vi "ProceduralControlSystem.vi"() -> ()   [LabVIEW 2021]
panel:
  out "Solenoid Outputs":bool[](array[boolean])
  in  "Sensor Values":dbl[](array[numeric])
  in  "File Path":path[](array[path])
  in  "Dry Test Run":bool
  in  "Ignition":bool
  in  "Mainain Pressure":bool
  in  "Device & Valve Diagnostics":bool[](array[boolean])
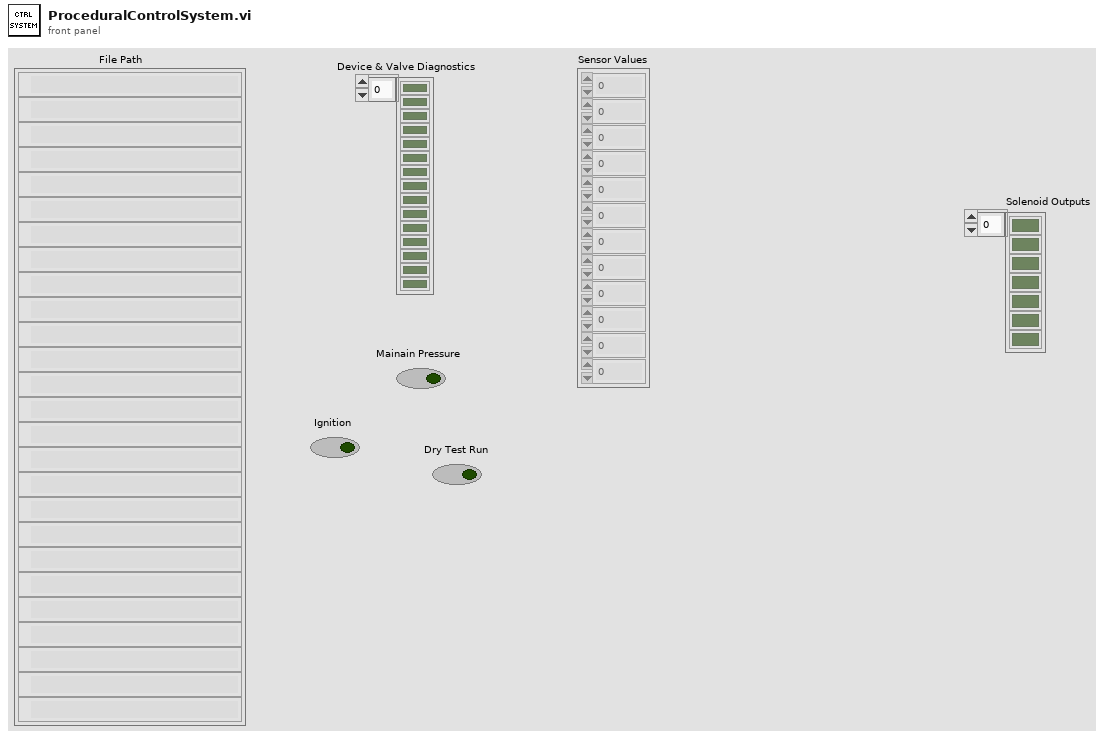
[diagram p1: front panel]
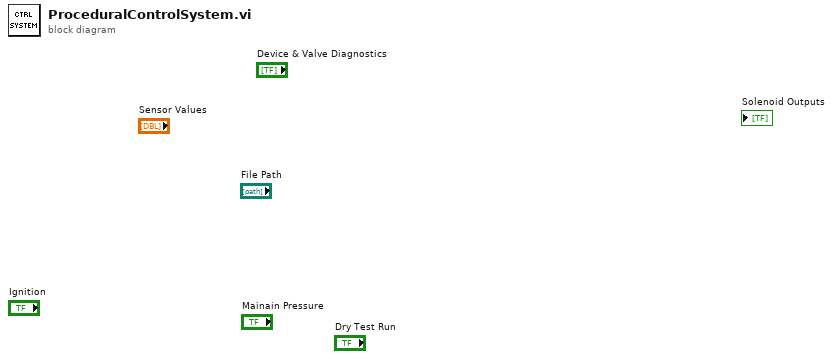
[diagram p0: block diagram]
diagram:
